vi "encoder_test_3mode_2motor_v2.vi"() -> ()   [LabVIEW 2014]
uses:
  <vilib>/eio/EIONode/EIONode.xnode
  <vilib>/rvi/FXPMathLib/FxpMul/XNode/nifxpmath_Multiplier.xnode
  <vilib>/rvi/FXPMathLib/sim/FxpSim.dll
  <vilib>/rvi/eio/common/nirviEmuTemplateMethod_errors.vi
  <vilib>/rvi/FXPMathLib/FxpSinAndCos/XNode/nifxpmath_SinAndCos.xnode
  <vilib>/rvi/FXPMathLib/FxpSinAndCos/simVIs/DllFxpSinAndCosTemp_sub.vi
  <vilib>/rvi/FXPMathLib/FxpSinAndCos/subVIs/nifxpmath_SinAndCos_SimConfig.ctl
  <vilib>/rvi/Analysis/measure/butterworth/XNode/niFpgaButterworthFilter.xnode
  <vilib>/rvi/FXPMathLib/FxpSub/XNode/nifxpmath_Sub.xnode
  <vilib>/rvi/FXPMathLib/FxpAdd/XNode/nifxpmath_Add.xnode
  <vilib>/rvi/DataTransferAndStorage/Container/XNode/niFpgaContainer.xnode
  <vilib>/rvi/interface/RandomDataEmulation/nirviRandomDataFpgaMultiElementTemplate.vi
panel:
  out "Dy_i":fxp<+/-,32,16>
  out "Dyr":fxp<+/-,64,32>
  in  "Direction_y":bool
  in  "Command type_y":i16(ring) items=["Step", "Ramp", "Sine"]
  out "Dy_error":fxp<+/-,57,33>
  out "Fmr_y":fxp<+/-,64,50>
  in  "Ki_y":fxp<+/-,16,1>
  in  "Dy_tolorence":fxp<+/-,18,1>
  in  "Kd_y":fxp<+/-,16,1>
  in  "Kp_y":fxp<+/-,16,1>
  in  "scaled coefficients_Dy_dd":i32[](array[numeric])=[780119100, 146811362]
  out "Dy_dd":fxp<+/-,36,47>
  out "va_y":fxp<+/-,36,7>
  out "vb_y":fxp<+/-,37,8>
  out "vd_y":fxp<+/-,20,5>
  out "vq_y":fxp<+/-,20,5> format="%.57g"
  in  "Stop motor_y":bool
  out "Dy_d (mm/s)":fxp<+,64,32>
  out "omega_y (rad/s)":fxp<+/-,64,35>
  in  "Velocity Estimation_y":i16(ring) items=["Step", "Ramp", "Sine"]
  out "Dy_d (T)":fxp<+/-,46,10>
  out "mt 2":u32
  out "omega_y (T)":fxp<+/-,20,9>
  out "omega_y (M)":fxp<+/-,64,30>
  out "Dy_d (M)":fxp<+/-,64,27>
  in  "Dy_d_M_Tc (mSec)":u32 format="%#_6f"
  out "omega_y(M_avg)":fxp<+/-,64,35>
  out "Dy_d (M_avg)":fxp<+,64,32>
  in  "Dy_d_M_avg_Tc (uSec)":u32 caption="Count(uSec)"
  out "rad_y(NrTheta)":fxp<+/-,48,33>
  out "Dy (mm)":fxp<+/-,56,32>
  out "Encoder Position_y":i32
  in  "Encoder Reset_y":bool
  out "omega_p (M_avg)":fxp<+/-,64,35>
  out "Dp_d (M_avg)":fxp<+/-,64,32>
  in  "Dp_d_M_avg_Tc (uSec)":u32 caption="D_d_M_avg_Tc (uSec)"
  out "omega_p (M)":fxp<+/-,64,30>
  out "Dp_d (M)":fxp<+/-,64,27>
  in  "Dp_d_M_Tc (mSec)":u32 format="%#_6f"
  out "Dp_d (T)":fxp<+/-,46,10>
  out "omega_p(T)":fxp<+/-,20,9>
  in  "Velocity Estimation_p":i16(ring) items=["M_avg method", "M method", "T method"]
  out "Dpr_ramp":fxp<+/-,64,30>
  out "Dpr_slope":fxp<+/-,33,17>
  in  "Dpr_time":fxp<+/-,16,11>
  out "Dpr_sin":fxp<+/-,28,11>
  out "Dpr_sin_d":fxp<+/-,64,16>
  out "Dpr_sin_dd":fxp<+/-,64,25>
  out "Sin omega_p":fxp<+/-,41,8>
  in  "Sin offset_p":fxp<+/-,27,10>
  in  "Sin magnitude_p":fxp<+/-,11,8>
  in  "Sin wave frequency_p (Hz)":fxp<+/-,21,5>
  out "Time now (s)":fxp<+,52,14>
  out "Dpr":fxp<+/-,64,31>
  in  "Dpr_end":fxp<+/-,16,11>
  in  "Command type_p":i16(ring) items=["Step", "Ramp", "Sine"]
  out "Dp_i":fxp<+/-,34,18>
  in  "Dp_tolorence":fxp<+/-,18,1>
  in  "Ki_p":fxp<+/-,20,6>
  out "Dp_error":fxp<+/-,24,11>
  in  "Direction_p":bool
  out "Fmr_p":fxp<+/-,64,31>
  in  "Kd_p":fxp<+/-,20,8>
  in  "Kp_p":fxp<+/-,20,12>
  in  "scaled coefficients_Dp_dd":i32[](array[numeric])=[780119100, 146811362]
  out "Dp_dd":fxp<+/-,36,29>
  in  "Ini coe.":bool
  out "va_p":fxp<+/-,38,8>
  out "vb_p":fxp<+/-,38,8>
  in  "Stop motor_p":bool
  out "vq_p":fxp<+/-,20,5> format="%.57g"
  out "vd_p":fxp<+/-,20,5>
  out "Dp_d (mm/s)":fxp<+/-,32,12>
  out "mt":u32
  out "omega_p (rad/s)":fxp<+/-,32,18>
  in  "mt0":u32
  out "Dp (mm)":fxp<+/-,22,7>
  out "rad_p(NrTheta)":fxp<+/-,33,18>
  out "Encoder Position_p":i32
  in  "Encoder Reset_p":bool
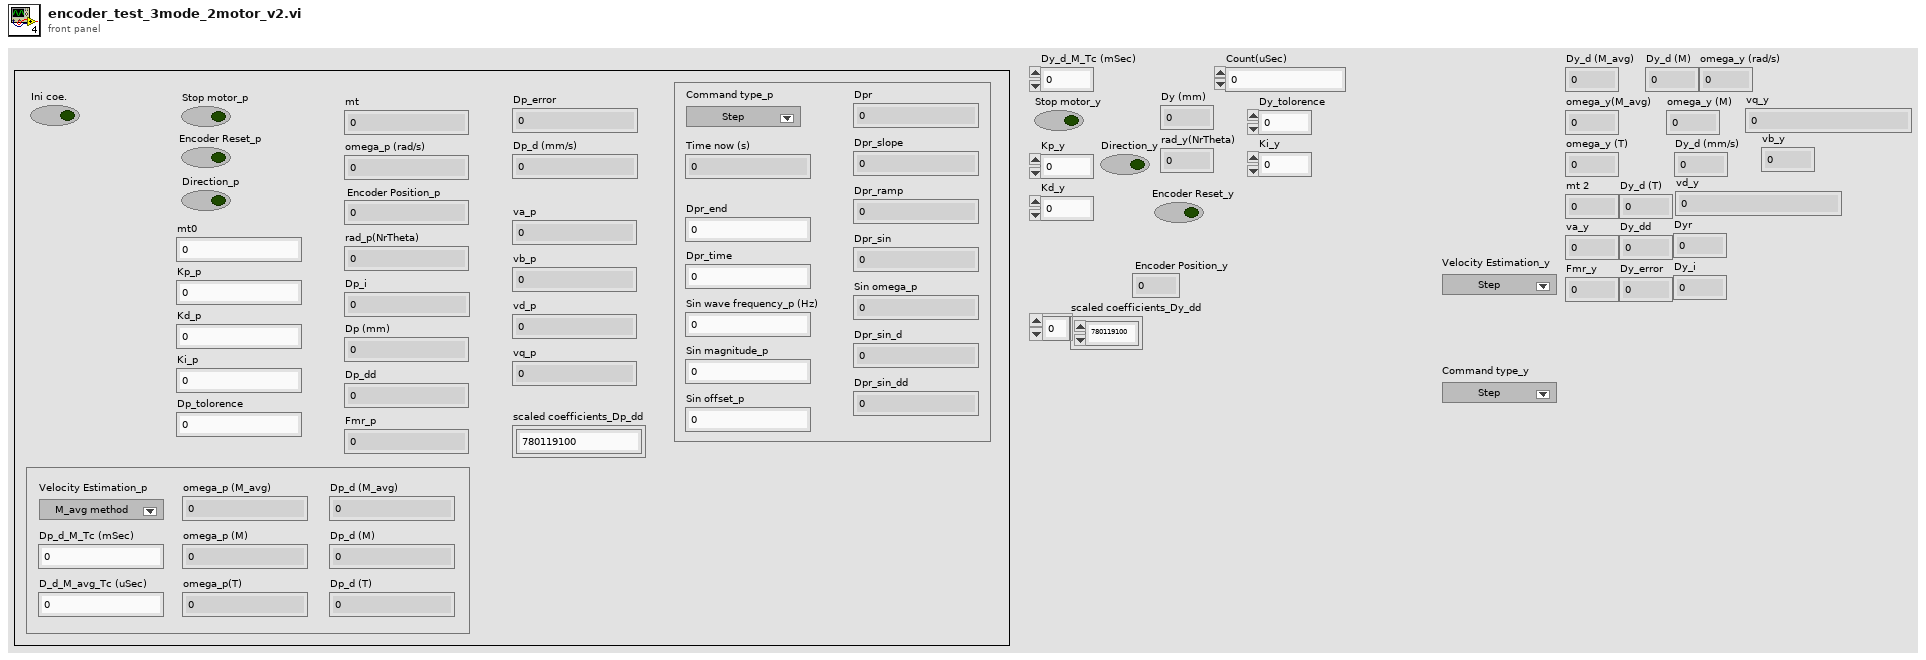
[diagram p1: front panel]
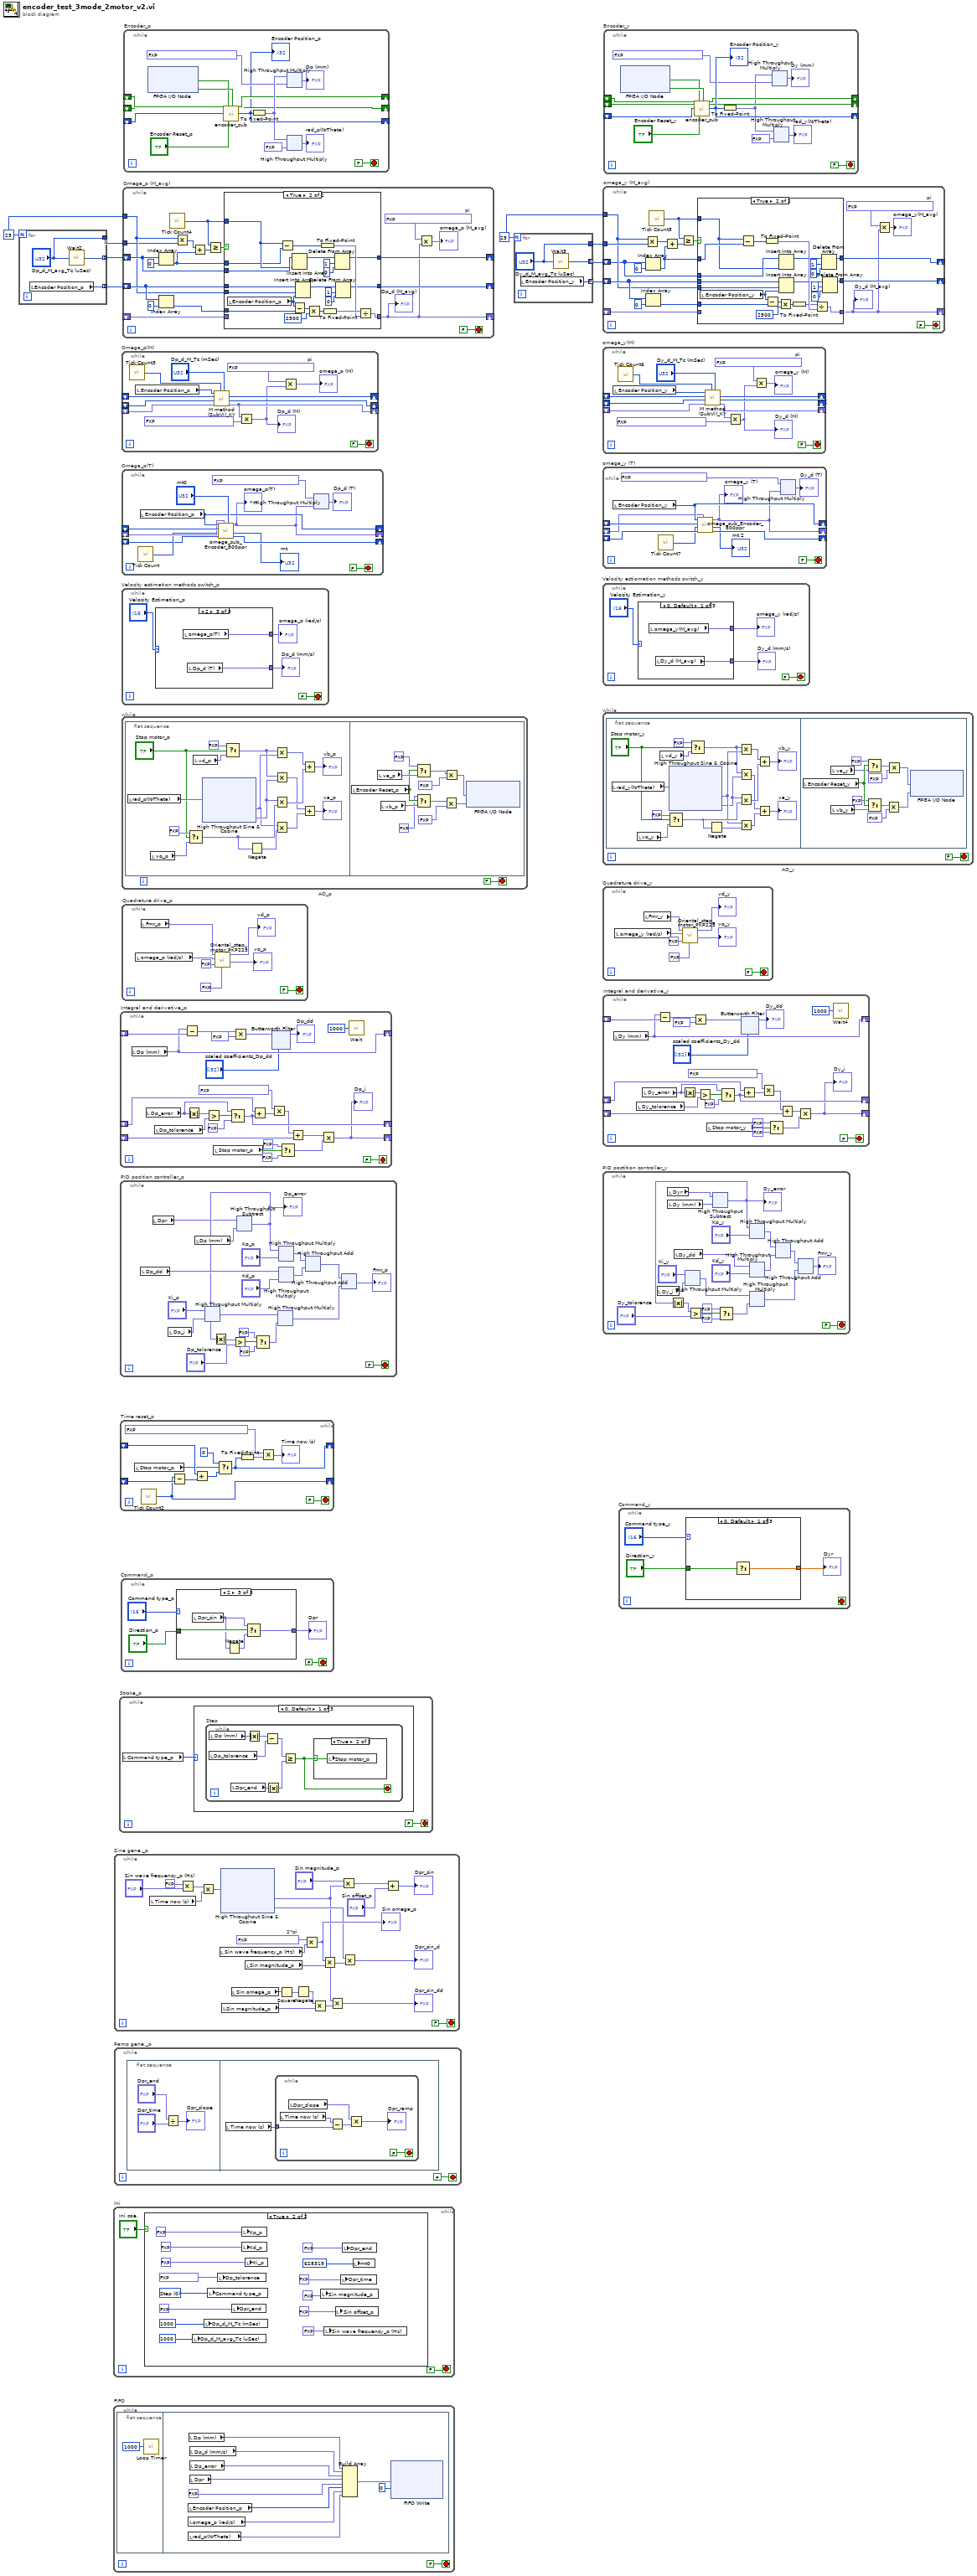
[diagram p0: block diagram]
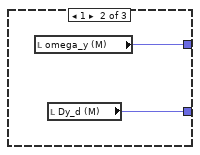
[diagram p4: hidden frame]
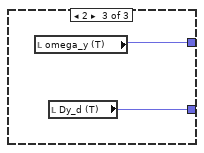
[diagram p5: hidden frame]
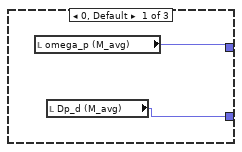
[diagram p8: hidden frame]
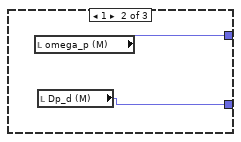
[diagram p9: hidden frame]
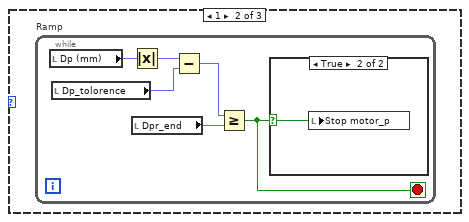
[diagram p11: hidden frame]
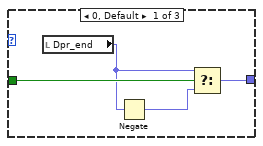
[diagram p14: hidden frame]
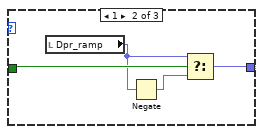
[diagram p15: hidden frame]
diagram:
  w4 = 25
  w8 = 25
  n1 = for {
    N: w8 -> [_]
    tunnel: ["Dp_d_M_avg_Tc (uSec)"] -> w5
    tunnel: [w10] -> w7 mode=indexing
    tunnel: [w9] -> w6 mode=indexing
    n2 = local read "Encoder Position_p"() -> (w9:i32)
    n3 = call "Wait2"("Count(uSec)"="Dp_d_M_avg_Tc (uSec)") -> ("Tick Count(uSec)"=w10:u32)
  }
  n4 = while "Ini" {
    stop <- FALSE stop-if-true
    n5 = case shown="True" "Ini coe." {
      frame False {
      }
      frame True {
        w21 = i16 0 items=["Step", "Ramp", "Sine"] ("Command type")
        n6 = local write "Dp_d_M_avg_Tc (uSec)"(u32 1000 ("D_d_M_avg_Tc (uSec)")) -> ()
        n7 = local write "Dp_d_M_Tc (mSec)"(u32 1000 ("D_d_M_Tc (uSec)")) -> ()
        n8 = local write "Command type_p"(w21) -> ()
        n9 = local write "Dp_tolorence"(fxp<+/-,14,3> 0.009765625 ("D_tolorence")) -> ()
        n10 = local write "Dpr_end"(fxp<+/-,16,11> 20.0 ("Dr_end")) -> ()
        n11 = local write "Kp_p"(fxp<+/-,20,12> 10.0 ("Kp")) -> ()
        n12 = local write "Kd_p"(fxp<+/-,20,8> 2.0 ("Kd")) -> ()
        n13 = local write "Ki_p"(fxp<+/-,20,6> 8.0 ("D_i")) -> ()
        n14 = local write "Sin magnitude_p"(fxp<+/-,11,8> 20.0 ("Sin magnitude")) -> ()
        n15 = local write "Sin wave frequency_p (Hz)"(fxp<+/-,21,5> 0.5 ("Sin wave frequency (Hz)")) -> ()
        n16 = local write "Sin offset_p"(fxp<+/-,27,10> 0.0 ("Sin offset")) -> ()
        n17 = local write "Dpr_time"(fxp<+/-,16,11> 5.0 ("Dr_time")) -> ()
        n18 = local write "Dpr_end"(fxp<+/-,11,7> 20.0 ("Fmr")) -> ()
        n19 = local write "mt0"(u32 628319 ("mt0")) -> ()
      }
    }
  }
  n20 = while "FIFO" {
    stop <- FALSE stop-if-true
    n21 = flat-sequence {
      frame #0 {
        n22 = call "Loop Timer"("Count(uSec)"=u32 1000) -> ()  [unwired: 1 out]
      }
      frame #1 {
        n23 = local read "Encoder Position_p"() -> (w33:i32)
        n24 = local read "omega_p (rad/s)"() -> (w32:fxp<+/-,32,18>)
        n25 = local read "rad_p(NrTheta)"() -> (w31:fxp<+/-,33,18>)
        n26 = local read "Dp (mm)"() -> (w37:fxp<+/-,22,7>)
        n27 = local read "Dp_d (mm/s)"() -> (w36:fxp<+/-,32,12>)
        n28 = local read "Dp_error"() -> (w35:fxp<+/-,24,11>)
        n29 = local read "Dpr"() -> (w34:fxp<+/-,64,31>)
        n30 = Build Array(w37, w36, w35, w34, fxp<+/-,64,32> 0.0 ("element"), w33, w32, w31) -> (w38:fxp<+/-,64,32>[])
        n31 = xnode ("FIFO Write")("Element"=w38, "Timeout"=0) -> ()  [unwired: 1 in, 2 out]
      }
    }
  }
  n32 = while "Sine gene._p" {
    stop <- FALSE stop-if-true
    w57 = fxp<+,20,3> 6.2831878662109375  # 2*pi
    n33 = local read "Time now (s)"() -> (w60:fxp<+,52,14>)
    n34 = Multiply(x=fxp<+,1,2> 2.0, y="Sin wave frequency_p (Hz)") -> (x*y=w61:fxp<+/-,21,6>)
    n35 = Multiply(x=w61, y=w60) -> (x*y=w41:fxp<+/-,64,20>)
    n36 = local read "Sin wave frequency_p (Hz)"() -> (w56:fxp<+/-,21,5>)
    n37 = xnode "High Throughput Sine & Cosine"("x (pi)"=w41) -> ("sin(x)"=w45:fxp<+/-,16,2>, "cos(x)"=w52:fxp<+/-,16,2>)
    n38 = local read "Sin magnitude_p"() -> (w47:fxp<+/-,11,8>)
    n39 = local read "Sin omega_p"() -> (w48:fxp<+/-,41,8>)
    n40 = local read "Sin magnitude_p"() -> (w51:fxp<+/-,11,8>)
    n41 = Square(x=w48) -> (x^2=w49:fxp<+,64,14>)
    n42 = Negate(x=w49) -> (-x=w46:fxp<+/-,64,15>)
    n43 = Multiply(x=w57, y=w56) -> (x*y=w53:fxp<+/-,41,8>)
    "Sin omega_p" <- w53
    n44 = Multiply(x=w46, y=w47) -> (x*y=w50:fxp<+/-,64,23>)
    n45 = Multiply(x=w53, y=w51) -> (x*y=w58:fxp<+/-,51,15>)
    n46 = Multiply(x=w45, y=w50) -> (x*y=→"Dpr_sin_dd":fxp<+/-,64,25>)
    n47 = Multiply(x="Sin magnitude_p", y=w45) -> (x*y=w59:fxp<+/-,27,10>)
    n48 = Multiply(x=w52, y=w58) -> (x*y=→"Dpr_sin_d":fxp<+/-,64,16>)
    n49 = Add(x=w59, y="Sin offset_p") -> (x+y=→"Dpr_sin":fxp<+/-,28,11>)
  }
  n50 = while "Ramp gene._p" {
    stop <- FALSE stop-if-true
    n51 = flat-sequence {
      frame #0 {
        n52 = Divide(x="Dpr_end", y="Dpr_time") -> (x/y=→"Dpr_slope":fxp<+/-,33,17>)
      }
      frame #1 {
        n53 = local read "Time now (s)"() -> (w98:fxp<+,52,14>)
        n54 = while {
          tunnel: w98 -> [w104]
          stop <- FALSE stop-if-true
          n55 = local read "Time now (s)"() -> (w101:fxp<+,52,14>)
          n56 = local read "Dpr_slope"() -> (w102:fxp<+/-,33,17>)
          n57 = Subtract(x=w101, y=w104) -> (x-y=w103:fxp<+/-,53,15>)
          n58 = Multiply(x=w102, y=w103) -> (x*y=→"Dpr_ramp":fxp<+/-,64,30>)
        }
      }
    }
  }
  n59 = while "Stroke_p" {
    stop <- FALSE stop-if-true
    n60 = local read "Command type_p"() -> (w106:i16)
    n61 = case shown="0, Default" w106 {
      frame 0, Default {
        n62 = while "Step" {
          stop <- w107 stop-if-true
          n63 = local read "Dp_tolorence"() -> (w109:fxp<+/-,18,1>)
          n64 = local read "Dp (mm)"() -> (w111:fxp<+/-,22,7>)
          n65 = local read "Dpr_end"() -> (w113:fxp<+/-,16,11>)
          n66 = Absolute Value(x=w111) -> (abs(x)=w110:fxp<+,22,7>)
          n67 = Subtract(x=w110, y=w109) -> (x-y=w108:fxp<+/-,25,8>)
          n68 = Absolute Value(x=w113) -> (abs(x)=w112:fxp<+,16,11>)
          n69 = Greater Or Equal?(x=w108, y=w112) -> (x >= y?=w107:bool)
          n70 = case shown="True" w107 {
            selector: w107 -> [_ w114]
            frame False {
            }
            frame True {
              n71 = local write "Stop motor_p"(w114) -> ()
            }
          }
        }
      }
      frame 1 {
        n72 = while "Ramp" {
          stop <- w115 stop-if-true
          n73 = local read "Dp (mm)"() -> (w117:fxp<+/-,22,7>)
          n74 = local read "Dp_tolorence"() -> (w119:fxp<+/-,18,1>)
          n75 = Absolute Value(x=w117) -> (abs(x)=w118:fxp<+,22,7>)
          n76 = local read "Dpr_end"() -> (w116:fxp<+/-,16,11>)
          n77 = Subtract(x=w118, y=w119) -> (x-y=w120:fxp<+/-,25,8>)
          n78 = Greater Or Equal?(x=w120, y=w116) -> (x >= y?=w115:bool)
          n79 = case shown="True" w115 {
            selector: w115 -> [_ w121]
            frame False {
            }
            frame True {
              n80 = local write "Stop motor_p"(w121) -> ()
            }
          }
        }
      }
      frame 2 {
      }
    }
  }
  n81 = while "Integral and derivative_p" {
    shift-right: [w142] -> _
    shift-left: _ -> [w146]
    shift-right: [w132] -> _
    shift-left: _ -> [w133]
    shift-right: [w122] -> _
    shift-left: _ -> [w126]
    stop <- FALSE stop-if-true
    n82 = local read "Dp (mm)"() -> (w142:fxp<+/-,22,7>)
    n83 = local read "Dp_error"() -> (w134:fxp<+/-,24,11>)
    n84 = local read "Dp_tolorence"() -> (w137:fxp<+/-,18,1>)
    n85 = Subtract(x=w142, y=w146) -> (x-y=w145:fxp<+/-,23,8>)
    n86 = Absolute Value(x=w134) -> (abs(x)=w138:fxp<+,24,11>)
    n87 = Greater?(x=w138, y=w137) -> (0:w136:bool)
    n88 = local read "Stop motor_p"() -> (w129:bool)
    n89 = Select(t=w134, s=w136, f=fxp<+,24,11> 0.0) -> (s? t:f=w132:fxp<+/-,25,12>)
    n90 = Multiply(x=w145, y=fxp<+/-,33,13> 1000.0) -> (x*y=w143:fxp<+/-,55,20>)
    n91 = Add(x=w133, y=w132) -> (x+y=w131:fxp<+/-,26,13>)
    n92 = Multiply(x=fxp<+/-,30,12> 0.000499725341796875, y=w131) -> (x*y=w125:fxp<+/-,55,24>)
    n93 = xnode "Butterworth Filter"("input data"=w143, "scaled coefficients"="scaled coefficients_Dp_dd") -> ("output data"=→"Dp_dd":fxp<+/-,36,24>)  [unwired: 1 in]
    n94 = Select(t=fxp<+,1,1> 0.0, s=w129, f=fxp<+,1,1> 1.0) -> (s? t:f=w123:fxp<+,1,1>)
    n95 = Add(x=w125, y=w126) -> (x+y=w124:fxp<+/-,32,16>)
    n96 = Multiply(x=w124, y=w123) -> (x*y=w122:fxp<+/-,32,16>)
    "Dp_i" <- w122
    n97 = call "Wait"("Count(uSec)"=u32 1000) -> ()  [unwired: 1 out]
  }
  n98 = while "PID position controller_p" {
    stop <- FALSE stop-if-true
    n99 = local read "Dp_dd"() -> (w172:fxp<+/-,36,29>)
    n100 = local read "Dpr"() -> (w156:fxp<+/-,64,31>)
    n101 = local read "Dp_i"() -> (w167:fxp<+/-,34,18>)
    n102 = local read "Dp (mm)"() -> (w176:fxp<+/-,22,7>)
    n103 = xnode ("High Throughput Multiply")("x"="Ki_p", "y"=w167) -> ("x*y"=w161:fxp<+/-,54,24>)
    n104 = xnode "High Throughput Subtract"("x"=w156, "y"=w176) -> ("x-y"=w165:fxp<+/-,64,32>)
    "Dp_error" <- w165
    n105 = Absolute Value(x=w165) -> (abs(x)=w166:fxp<+,64,32>)
    n106 = Greater?(x=w166, y="Dp_tolorence") -> (0:w164:bool)
    n107 = Select(t=fxp<+,10,2> 1.0, s=w164, f=fxp<+,10,2> 0.0) -> (s? t:f=w160:fxp<+,10,2>)
    n108 = xnode ("High Throughput Multiply")("x"=w161, "y"=w160) -> ("x*y"=w157:fxp<+/-,64,26>)
    n109 = xnode ("High Throughput Multiply")("x"=w165, "y"="Kp_p") -> ("x*y"=w174:fxp<+/-,64,44>)
    n110 = xnode ("High Throughput Multiply")("x"=w172, "y"="Kd_p") -> ("x*y"=w173:fxp<+/-,56,37>)
    n111 = xnode ("High Throughput Add")("x"=w174, "y"=w173) -> ("x+y"=w158:fxp<+/-,64,45>)
    n112 = xnode ("High Throughput Add")("x"=w158, "y"=w157) -> ("x+y"=→"Fmr_p":fxp<+/-,64,46>)
  }
  n113 = while "Time reset_p" {
    shift-right: [w180] -> _
    shift-left: _ -> [w187]
    shift-right: [w182] -> _
    shift-left: _ -> [w183]
    stop <- FALSE stop-if-true
    n114 = local read "Stop motor_p"() -> (w185:bool)
    n115 = call "Tick Count2"() -> ("Tick Count(uSec)"=w182:u32)
    n116 = Subtract(x=w182, y=w183) -> (x-y=w188:u32)
    n117 = Add(x=w187, y=w188) -> (x+y=w186:u32)
    n118 = Select(t=u32 0, s=w185, f=w186) -> (s? t:f=w180:u32)
    n119 = To Fixed-Point(number=w180) -> (fixed-point=w179:fxp<+,32,32>)  [unwired: 1 in]
    n120 = Multiply(x=fxp<+,20,-18> 1.0000003385357559e-06, y=w179) -> (x*y=→"Time now (s)":fxp<+,52,14>)
  }
  n121 = while "Command_p" {
    stop <- FALSE stop-if-true
    n122 = case shown="2" "Command type_p" {
      tunnel: [w193 w197 w201] -> w191
      tunnel: "Direction_p" -> [w196 w200 w204]
      frame 0, Default {
        n123 = local read "Dpr_end"() -> (w195:fxp<+/-,16,11>)
        n124 = Negate(x=w195) -> (-x=w194:fxp<+/-,17,12>)
        n125 = Select(t=w195, s=w196, f=w194) -> (s? t:f=w193:fxp<+/-,17,12>)
      }
      frame 1 {
        n126 = local read "Dpr_ramp"() -> (w198:fxp<+/-,64,30>)
        n127 = Negate(x=w198) -> (-x=w199:fxp<+/-,64,31>)
        n128 = Select(t=w198, s=w200, f=w199) -> (s? t:f=w197:fxp<+/-,64,31>)
      }
      frame 2 {
        n129 = local read "Dpr_sin"() -> (w202:fxp<+/-,28,11>)
        n130 = Negate(x=w202) -> (-x=w203:fxp<+/-,27,10>)
        n131 = Select(t=w202, s=w204, f=w203) -> (s? t:f=w201:fxp<+/-,28,11>)
      }
    }
    "Dpr" <- w191
  }
  n132 = while "Omega_p(M)" {
    shift-right: [w216] -> _
    shift-left: _ -> [w217]
    shift-right: [w212] -> _
    shift-left: _ -> [w213]
    shift-right: [w210] -> _
    shift-left: _ -> [w211]
    stop <- FALSE stop-if-true
    w207 = fxp<+/-,27,3> 3.1415926218032837  # pi
    n133 = call "Tick Count3"() -> ("Tick Count(mSec)"=w215:u32)
    n134 = local read "Encoder Position_p"() -> (w218:i32)
    n135 = call "M method (SubVI)_KY.vi"("Tc (mSec)"="Dp_d_M_Tc (mSec)", "Tick Count (mSec)"=w215, "Encoder velocity_pre (pulse/s)"=w211, "Shift Register in 2"=w213, "Shift Register in 1"=w217, "Encoder pulses"=w218) -> ("Encoder velocity (pulse/s)"=w210:fxp<+/-,64,32>, "Shift Register out 2"=w212:i32, "Shift Register out 1"=w216:u32)  [unwired: 3 in]
    n136 = Multiply(x=w210, y=fxp<+/-,20,-5> 0.002499997615814209) -> (x*y=w208:fxp<+/-,64,27>)
    "Dp_d (M)" <- w208
    n137 = Multiply(x=w207, y=w208) -> (x*y=→"omega_p (M)":fxp<+/-,64,30>)
  }
  n138 = while "Omega_p(T)" {
    shift-right: [w228] -> _
    shift-left: _ -> [w229]
    shift-right: [w221] -> _
    shift-left: _ -> [w227]
    shift-right: [w224] -> _
    shift-left: _ -> [w225]
    stop <- FALSE stop-if-true
    n139 = call "Tick Count"() -> ("Tick Count(Ticks)"=w226:u32)
    n140 = local read "Encoder Position_p"() -> (w228:i32)
    n141 = call "omega_sub_Encoder_800ppr.vi"("mt0"="mt0", "omega_pre"=w227, "ticks_m_pre"=w225, "ticks"=w226, "count_pre"=w229, "count"=w228) -> ("ticks_m"=w224:u32, "mt"=→"mt":u32, "omega"=w221:fxp<+/-,20,9>)  [unwired: 3 in]
    "omega_p(T)" <- w221
    n142 = xnode ("High Throughput Multiply")("x"=fxp<+/-,26,1> 0.3183099031448364, "y"=w221) -> ("x*y"=→"Dp_d (T)":fxp<+/-,46,10>)
  }
  n143 = while "Velocity estimation methods switch_p" {
    stop <- FALSE stop-if-true
    n144 = case shown="2" "Velocity Estimation_p" {
      tunnel: [w236 w238 w240] -> w233
      tunnel: [w235 w237 w239] -> w232
      frame 0, Default {
        n145 = local read "omega_p (M_avg)"() -> (w236:fxp<+/-,64,35>)
        n146 = local read "Dp_d (M_avg)"() -> (w235:fxp<+/-,64,32>)
      }
      frame 1 {
        n147 = local read "omega_p (M)"() -> (w238:fxp<+/-,64,30>)
        n148 = local read "Dp_d (M)"() -> (w237:fxp<+/-,64,27>)
      }
      frame 2 {
        n149 = local read "omega_p(T)"() -> (w240:fxp<+/-,20,9>)
        n150 = local read "Dp_d (T)"() -> (w239:fxp<+/-,46,10>)
      }
    }
    "Dp_d (mm/s)" <- w232
    "omega_p (rad/s)" <- w233
  }
  n151 = while "AO_p" {
    stop <- FALSE stop-if-true
    n152 = flat-sequence {
      frame #0 {
        n153 = local read "rad_p(NrTheta)"() -> (w257:fxp<+/-,33,18>)
        n154 = local read "vq_p"() -> (w255:fxp<+/-,20,5>)
        n155 = Select(t=fxp<+,20,5> 0.0, s="Stop motor_p", f=w255) -> (s? t:f=w252:fxp<+/-,21,6>)
        n156 = local read "vd_p"() -> (w256:fxp<+/-,20,5>)
        n157 = xnode "High Throughput Sine & Cosine"("x (pi)"=w257) -> ("sin(x)"=w248:fxp<+/-,17,2>, "cos(x)"=w250:fxp<+/-,17,2>)
        n158 = Select(t=fxp<+,20,5> 0.0, s="Stop motor_p", f=w256) -> (s? t:f=w249:fxp<+/-,21,6>)
        n159 = Negate(x=w252) -> (-x=w251:fxp<+/-,21,6>)
        n160 = Multiply(x=w249, y=w248) -> (x*y=w247:fxp<+/-,37,7>)
        n161 = Multiply(x=w249, y=w250) -> (x*y=w245:fxp<+/-,37,7>)
        n162 = Multiply(x=w250, y=w252) -> (x*y=w246:fxp<+/-,37,7>)
        n163 = Multiply(x=w248, y=w251) -> (x*y=w244:fxp<+/-,37,7>)
        n164 = Add(x=w247, y=w246) -> (x+y=→"vb_p":fxp<+/-,38,8>)
        n165 = Add(x=w245, y=w244) -> (x+y=→"va_p":fxp<+/-,38,8>)
      }
      frame #1 {
        n166 = local read "Encoder Reset_p"() -> (w291:bool)
        n167 = local read "va_p"() -> (w293:fxp<+/-,38,8>)
        n168 = local read "vb_p"() -> (w292:fxp<+/-,38,8>)
        n169 = Select(t=fxp<+/-,20,5> 5.0 ("y"), s=w291, f=w293) -> (s? t:f=w294:fxp<+/-,38,8>)
        n170 = Select(t=fxp<+/-,20,5> 0.0 ("y"), s=w291, f=w292) -> (s? t:f=w295:fxp<+/-,38,8>)
        n171 = Multiply(x=w295, y=fxp<+/-,20,5> -0.5) -> (x*y=w299:fxp<+/-,57,12>)
        n172 = Multiply(x=w294, y=fxp<+/-,20,5> -0.5) -> (x*y=w298:fxp<+/-,57,12>)
        n173 = xnode "FPGA I/O Node"("Mod8/AO0"=w298, "Mod8/AO1"=w299) -> ()  [unwired: 2 in, 2 out]
      }
    }
  }
  n174 = while "Quadrature drive_p" {
    stop <- FALSE stop-if-true
    n175 = local read "omega_p (rad/s)"() -> (w302:fxp<+/-,32,18>)
    n176 = local read "Fmr_p"() -> (w300:fxp<+/-,64,31>)
    n177 = call "Oriental_step_motor_PKP225.vi"("F_Threshold"=fxp<+,12,12> 10.0, "dFmr"=fxp<+/-,25,15> 0.0, "omega"=w302, "Fmr"=w300) -> ("vq_F"=→"vq_p":fxp<+/-,20,5>, "vd_F"=→"vd_p":fxp<+/-,20,5>)  [unwired: 6 in]
  }
  n178 = while "Omega_p (M_avg)" {
    tunnel: w8 -> [w318]
    shift-right: [w311] -> _
    shift-left: w7 -> [w322]
    shift-right: [w310] -> _
    shift-left: _ -> [w313]
    shift-right: [w312] -> _
    shift-left: w6 -> [w321]
    tunnel: w5 -> [w315]
    stop <- FALSE stop-if-true
    w309 = fxp<+/-,27,3> 3.1415926218032837  # pi
    n179 = Index Array(array=w322, index=0) -> (element=w316:u32)
    n180 = Index Array(array=w321, index=0) -> (element=w317:i32)
    n181 = call "Tick Count4"() -> ("Tick Count(uSec)"=w319:u32)
    n182 = Multiply(x=w318, y=w315) -> (x*y=w323:u32)
    n183 = Add(x=w323, y=w316) -> (x+y=w320:u32)
    n184 = Greater Or Equal?(x=w319, y=w320) -> (x >= y?=w314:bool)
    n185 = case shown="True" w314 {
      tunnel: w322 -> [w328 w345]
      tunnel: w321 -> [w327 w344]
      tunnel: w319 -> [_ w337]
      tunnel: w318 -> [_ w343]
      tunnel: w317 -> [_ w341]
      tunnel: w316 -> [_ w336]
      tunnel: w313 -> [w326 _]
      tunnel: [w327 w331] -> w312
      tunnel: [w328 w330] -> w311
      tunnel: [w326 w329] -> w310
      frame False {
      }
      frame True {
        n186 = local read "Encoder Position_p"() -> (w342:i32)
        n187 = Subtract(x=w337, y=w336) -> (x-y=w334:u32)
        n188 = Insert Into Array(array=w345, new element=w337) -> (w346:u32[])  [unwired: 1 in]
        n189 = Subtract(x=w342, y=w341) -> (x-y=w340:i32)
        n190 = Insert Into Array(array=w344, index=w343, new element=w342) -> (w347:i32[])
        n191 = Multiply(x=w340, y=2500) -> (x*y=w338:i32)
        n192 = To Fixed-Point(number=w334) -> (fixed-point=w332:fxp<+,32,32>)  [unwired: 1 in]
        n193 = To Fixed-Point(number=w338) -> (fixed-point=w333:fxp<+/-,32,32>)  [unwired: 1 in]
        n194 = Delete From Array(array=w346, length=1, index=0) -> (array with subset deleted=w330:u32[])  [unwired: 1 out]
        n195 = Delete From Array(array=w347, length=1, index=0) -> (array with subset deleted=w331:i32[])  [unwired: 1 out]
        n196 = Divide(x=w333, y=w332) -> (x/y=w329:fxp<+/-,64,32>)
      }
    }
    "Dp_d (M_avg)" <- w310
    n197 = Multiply(x=w309, y=w310) -> (x*y=→"omega_p (M_avg)":fxp<+/-,64,35>)
  }
  n198 = while "Encoder_p" {
    shift-right: [w357] -> _
    shift-left: _ -> [w359]
    shift-right: [w356] -> _
    shift-left: _ -> [w358]
    shift-right: [w354] -> _
    shift-left: _ -> [w355]
    stop <- FALSE stop-if-true
    n199 = xnode "FPGA I/O Node"() -> ("Mod4/DI3"=w364:bool, "Mod4/DI4"=w365:bool)  [unwired: 2 in, 2 out]
    n200 = call "encoder_sub.vi"("A_pre"=w359, "B_pre"=w358, "Encoder Position_pre"=w355, "A input"=w364, "Encoder Position Reset"="Encoder Reset_p", "B input"=w365) -> ("A"=w357:bool, "B"=w356:bool, "Encoder Position (Counts)"=w354:i32)  [unwired: 19 in]
    "Encoder Position_p" <- w354
    n201 = To Fixed-Point(number=w354) -> (fixed-point=w362:fxp<+/-,32,32>)  [unwired: 1 in]
    n202 = xnode ("High Throughput Multiply")("x"=w362, "y"=fxp<+/-,24,0> 0.002499997615814209) -> ("x*y"=→"Dp (mm)":fxp<+/-,56,32>)
    n203 = xnode ("High Throughput Multiply")("x"=w362, "y"=fxp<+/-,24,0> 0.125) -> ("x*y"=→"rad_p(NrTheta)":fxp<+/-,56,32>)
  }
  n204 = for {
    N: w4 -> [_]
    tunnel: ["Dy_d_M_avg_Tc (uSec)"] -> w3
    tunnel: [w367] -> w1 mode=indexing
    tunnel: [w366] -> w2 mode=indexing
    n205 = local read "Encoder Position_y"() -> (w366:i32)
    n206 = call "Wait3"("Count(uSec)"="Dy_d_M_avg_Tc (uSec)") -> ("Tick Count(uSec)"=w367:u32)
  }
  n207 = while "omega_y(M)" {
    shift-right: [w375] -> _
    shift-left: _ -> [w379]
    shift-right: [w376] -> _
    shift-left: _ -> [w378]
    shift-right: [w374] -> _
    shift-left: _ -> [w377]
    stop <- FALSE stop-if-true
    w371 = fxp<+/-,27,3> 3.1415926218032837  # pi
    n208 = local read "Encoder Position_y"() -> (w382:i32)
    n209 = call "Tick Count6"() -> ("Tick Count(mSec)"=w381:u32)
    n210 = call "M method (SubVI)_KY.vi"("Tc (mSec)"="Dy_d_M_Tc (mSec)", "Tick Count (mSec)"=w381, "Encoder velocity_pre (pulse/s)"=w377, "Shift Register in 2"=w378, "Shift Register in 1"=w379, "Encoder pulses"=w382) -> ("Encoder velocity (pulse/s)"=w374:fxp<+/-,64,32>, "Shift Register out 2"=w376:i32, "Shift Register out 1"=w375:u32)  [unwired: 3 in]
    n211 = Multiply(x=w374, y=fxp<+/-,20,-5> 0.002499997615814209) -> (x*y=w372:fxp<+/-,64,27>)
    "Dy_d (M)" <- w372
    n212 = Multiply(x=w371, y=w372) -> (x*y=→"omega_y (M)":fxp<+/-,64,30>)
  }
  n213 = while "omega_y (T)" {
    shift-right: [w392] -> _
    shift-left: _ -> [w391]
    shift-right: [w386] -> _
    shift-left: _ -> [w390]
    shift-right: [w393] -> _
    shift-left: _ -> [w389]
    stop <- FALSE stop-if-true
    n214 = local read "Encoder Position_y"() -> (w392:i32)
    n215 = call "Tick Count7"() -> ("Tick Count(Ticks)"=w388:u32)
    n216 = call "omega_sub_Encoder_800ppr.vi"("omega_pre"=w390, "ticks_m_pre"=w389, "ticks"=w388, "count_pre"=w391, "count"=w392) -> ("ticks_m"=w393:u32, "mt"=→"mt 2":u32, "omega"=w386:fxp<+/-,20,9>)  [unwired: 4 in]
    "omega_y (T)" <- w386
    n217 = xnode "High Throughput Multiply"("x"=fxp<+/-,26,1> 0.3183099031448364, "y"=w386) -> ("x*y"=→"Dy_d (T)":fxp<+/-,46,10>)
  }
  n218 = while "Velocity estiomation methods switch_y" {
    stop <- FALSE stop-if-true
    n219 = case shown="0, Default" "Velocity Estimation_y" {
      tunnel: [w399 w400 w403] -> w396
      tunnel: [w398 w401 w402] -> w395
      frame 0, Default {
        n220 = local read "omega_y(M_avg)"() -> (w399:fxp<+/-,64,35>)
        n221 = local read "Dy_d (M_avg)"() -> (w398:fxp<+,64,32>)
      }
      frame 1 {
        n222 = local read "omega_y (M)"() -> (w400:fxp<+/-,64,30>)
        n223 = local read "Dy_d (M)"() -> (w401:fxp<+/-,64,27>)
      }
      frame 2 {
        n224 = local read "omega_y (T)"() -> (w403:fxp<+/-,20,9>)
        n225 = local read "Dy_d (T)"() -> (w402:fxp<+/-,46,10>)
      }
    }
    "omega_y (rad/s)" <- w396
    "Dy_d (mm/s)" <- w395
  }
  n226 = while "AO_y" {
    stop <- FALSE stop-if-true
    n227 = flat-sequence {
      frame #0 {
        n228 = local read "rad_y(NrTheta)"() -> (w416:fxp<+/-,48,33>)
        n229 = local read "vq_y"() -> (w419:fxp<+/-,20,5>)
        n230 = local read "vd_y"() -> (w418:fxp<+/-,20,5>)
        n231 = xnode "High Throughput Sine & Cosine"("x (pi)"=w416) -> ("sin(x)"=w412:fxp<+/-,16,2>, "cos(x)"=w411:fxp<+/-,16,2>)
        n232 = Select(t=fxp<+,1,1> 0.0, s="Stop motor_y", f=w419) -> (s? t:f=w414:fxp<+/-,20,5>)
        n233 = Select(t=fxp<+/-,20,5> 0.0, s="Stop motor_y", f=w418) -> (s? t:f=w413:fxp<+/-,20,5>)
        n234 = Negate(x=w414) -> (-x=w415:fxp<+/-,21,6>)
        n235 = Multiply(x=w413, y=w412) -> (x*y=w410:fxp<+/-,36,7>)
        n236 = Multiply(x=w413, y=w411) -> (x*y=w408:fxp<+/-,36,7>)
        n237 = Multiply(x=w411, y=w414) -> (x*y=w409:fxp<+/-,36,7>)
        n238 = Multiply(x=w412, y=w415) -> (x*y=w407:fxp<+/-,35,6>)
        n239 = Add(x=w410, y=w409) -> (x+y=→"vb_y":fxp<+/-,37,8>)
        n240 = Add(x=w408, y=w407) -> (x+y=→"va_y":fxp<+/-,36,7>)
      }
      frame #1 {
        n241 = local read "Encoder Reset_y"() -> (w462:bool)
        n242 = local read "va_y"() -> (w461:fxp<+/-,36,7>)
        n243 = local read "vb_y"() -> (w460:fxp<+/-,37,8>)
        n244 = Select(t=fxp<+/-,20,5> 5.0, s=w462, f=w461) -> (s? t:f=w457:fxp<+/-,36,7>)
        n245 = Select(t=fxp<+/-,20,5> 0.0, s=w462, f=w460) -> (s? t:f=w456:fxp<+/-,37,8>)
        n246 = Multiply(x=w456, y=fxp<+/-,20,5> -0.5) -> (x*y=w452:fxp<+/-,55,11>)
        n247 = Multiply(x=w457, y=fxp<+/-,20,5> -0.5) -> (x*y=w453:fxp<+/-,55,11>)
        n248 = xnode "FPGA I/O Node"("Mod8/AO2"=w453, "Mod8/AO3"=w452) -> ()  [unwired: 2 in, 2 out]
      }
    }
  }
  n249 = while "Quadrature drive_y" {
    stop <- FALSE stop-if-true
    n250 = local read "omega_y (rad/s)"() -> (w469:fxp<+/-,64,35>)
    n251 = local read "Fmr_y"() -> (w464:fxp<+/-,64,50>)
    n252 = call "Oriental_step_motor_PKP225.vi"("F_Threshold"=fxp<+,12,12> 10.0, "dFmr"=fxp<+/-,25,15> 0.0, "omega"=w469, "Fmr"=w464) -> ("vq_F"=→"vq_y":fxp<+/-,20,5>, "vd_F"=→"vd_y":fxp<+/-,20,5>)  [unwired: 6 in]
  }
  n253 = while "PID postition controller_y" {
    stop <- FALSE stop-if-true
    n254 = local read "Dy_i"() -> (w471:fxp<+/-,32,16>)
    n255 = local read "Dyr"() -> (w472:fxp<+/-,64,32>)
    n256 = local read "Dy (mm)"() -> (w481:fxp<+/-,56,32>)
    n257 = local read "Dy_dd"() -> (w482:fxp<+/-,36,47>)
    n258 = xnode "High Throughput Multiply"("x"="Ki_y", "y"=w471) -> ("x*y"=w480:fxp<+/-,48,17>)
    n259 = xnode "High Throughput Subtract"("x"=w472, "y"=w481) -> ("x-y"=w473:fxp<+/-,64,33>)
    "Dy_error" <- w473
    n260 = Absolute Value(x=w473) -> (abs(x)=w474:fxp<+,64,33>)
    n261 = Greater?(x=w474, y="Dy_tolorence") -> (0:w485:bool)
    n262 = Select(t=fxp<+,1,1> 1.0, s=w485, f=fxp<+,1,1> 0.0) -> (s? t:f=w488:fxp<+,1,1>)
    n263 = xnode "High Throughput Multiply"("x"=w473, "y"="Kp_y") -> ("x*y"=w479:fxp<+/-,64,34>)
    n264 = xnode "High Throughput Multiply"("x"=w482, "y"="Kd_y") -> ("x*y"=w478:fxp<+/-,52,48>)
    n265 = xnode "High Throughput Multiply"("x"=w480, "y"=w488) -> ("x*y"=w476:fxp<+/-,48,17>)
    n266 = xnode "High Throughput Add"("x"=w479, "y"=w478) -> ("x+y"=w477:fxp<+/-,64,49>)
    n267 = xnode "High Throughput Add"("x"=w477, "y"=w476) -> ("x+y"=→"Fmr_y":fxp<+/-,64,50>)
  }
  n268 = while "omega_y (M_avg)" {
    tunnel: w4 -> [w500]
    tunnel: w3 -> [w506]
    shift-right: [w496] -> _
    shift-left: w1 -> [w497]
    shift-right: [w495] -> _
    shift-left: w2 -> [w501]
    shift-right: [w493] -> _
    shift-left: _ -> [w498]
    stop <- FALSE stop-if-true
    w494 = fxp<+/-,27,3> 3.1415926218032837  # pi
    n269 = Multiply(x=w500, y=w506) -> (x*y=w505:u32)
    n270 = Index Array(array=w497, index=0) -> (element=w502:u32)
    n271 = Index Array(array=w501, index=0) -> (element=w499:i32)
    n272 = call "Tick Count5"() -> ("Tick Count(uSec)"=w503:u32)
    n273 = Add(x=w505, y=w502) -> (x+y=w509:u32)
    n274 = Greater Or Equal?(x=w503, y=w509) -> (x >= y?=w504:bool)
    n275 = case shown="True" w504 {
      tunnel: w503 -> [_ w532]
      tunnel: w502 -> [_ w533]
      tunnel: w501 -> [w511 w522]
      tunnel: w500 -> [_ w523]
      tunnel: w499 -> [_ w524]
      tunnel: w498 -> [w510 _]
      tunnel: w497 -> [w512 w534]
      tunnel: [w512 w515] -> w496
      tunnel: [w511 w514] -> w495
      tunnel: [w510 w513] -> w493
      frame False {
      }
      frame True {
        n276 = local read "Encoder Position_y"() -> (w525:i32)
        n277 = Subtract(x=w532, y=w533) -> (x-y=w531:u32)
        n278 = To Fixed-Point(number=w531) -> (fixed-point=w530:fxp<+,32,32>)  [unwired: 1 in]
        n279 = Subtract(x=w525, y=w524) -> (x-y=w526:i32)
        n280 = Multiply(x=w526, y=u32 2500) -> (x*y=w528:u32)
        n281 = Insert Into Array(array=w534, new element=w532) -> (w520:u32[])  [unwired: 1 in]
        n282 = Insert Into Array(array=w522, index=w523, new element=w525) -> (w521:i32[])
        n283 = To Fixed-Point(number=w528) -> (fixed-point=w529:fxp<+,32,32>)  [unwired: 1 in]
        n284 = Divide(x=w529, y=w530) -> (x/y=w513:fxp<+,64,32>)
        n285 = Delete From Array(array=w520, length=1, index=0) -> (array with subset deleted=w515:u32[])  [unwired: 1 out]
        n286 = Delete From Array(array=w521, length=1, index=0) -> (array with subset deleted=w514:i32[])  [unwired: 1 out]
      }
    }
    "Dy_d (M_avg)" <- w493
    n287 = Multiply(x=w494, y=w493) -> (x*y=→"omega_y(M_avg)":fxp<+/-,64,35>)
  }
  n288 = while "Integral and derivative_y" {
    shift-right: [w556] -> _
    shift-left: _ -> [w559]
    shift-right: [w545] -> _
    shift-left: _ -> [w536]
    shift-right: [w538] -> _
    shift-left: _ -> [w537]
    stop <- FALSE stop-if-true
    n289 = local read "Dy (mm)"() -> (w556:fxp<+/-,56,32>)
    n290 = local read "Dy_tolorence"() -> (w551:fxp<+/-,18,1>)
    n291 = local read "Dy_error"() -> (w548:fxp<+/-,57,33>)
    n292 = Subtract(x=w556, y=w559) -> (x-y=w558:fxp<+/-,57,33>)
    n293 = Absolute Value(x=w548) -> (abs(x)=w552:fxp<+,57,33>)
    n294 = Multiply(x=w558, y=fxp<+,7,10> 1000.0) -> (x*y=w555:fxp<+/-,64,43>)
    n295 = Greater?(x=w552, y=w551) -> (0:w550:bool)
    n296 = local read "Stop motor_y"() -> (w542:bool)
    n297 = Select(t=w548, s=w550, f=fxp<+,24,11> 0.0) -> (s? t:f=w545:fxp<+/-,57,33>)
    n298 = xnode "Butterworth Filter"("input data"=w555, "scaled coefficients"="scaled coefficients_Dy_dd") -> ("output data"=→"Dy_dd":fxp<+/-,36,47>)  [unwired: 1 in]
    n299 = Add(x=w536, y=w545) -> (x+y=w547:fxp<+/-,58,34>)
    n300 = Multiply(x=fxp<+/-,30,12> 0.000499725341796875, y=w547) -> (x*y=w544:fxp<+/-,64,46>)
    n301 = Select(t=fxp<+,1,1> 0.0, s=w542, f=fxp<+,1,1> 1.0) -> (s? t:f=w539:fxp<+,1,1>)
    n302 = Add(x=w544, y=w537) -> (x+y=w543:fxp<+/-,32,16>)
    n303 = Multiply(x=w543, y=w539) -> (x*y=w538:fxp<+/-,32,16>)
    "Dy_i" <- w538
    n304 = call "Wait4"("Count(uSec)"=u32 1000) -> ()  [unwired: 1 out]
  }
  n305 = while "Encoder_y" {
    shift-right: [w577] -> _
    shift-left: _ -> [w575]
    shift-right: [w578] -> _
    shift-left: _ -> [w576]
    shift-right: [w581] -> _
    shift-left: _ -> [w580]
    stop <- FALSE stop-if-true
    n306 = xnode "FPGA I/O Node"() -> ("Mod4/DI0"=w582:bool, "Mod4/DI1"=w583:bool)  [unwired: 2 in, 2 out]
    n307 = call "encoder_sub.vi"("A_pre"=w575, "B_pre"=w576, "Encoder Position_pre"=w580, "A input"=w582, "Encoder Position Reset"="Encoder Reset_y", "B input"=w583) -> ("A"=w577:bool, "B"=w578:bool, "Encoder Position (Counts)"=w581:i32)  [unwired: 19 in]
    "Encoder Position_y" <- w581
    n308 = To Fixed-Point(number=w581) -> (fixed-point=w572:fxp<+/-,32,32>)  [unwired: 1 in]
    n309 = xnode "High Throughput Multiply"("x"=w572, "y"=fxp<+/-,24,0> 0.002499997615814209) -> ("x*y"=→"Dy (mm)":fxp<+/-,56,32>)
    n310 = xnode "High Throughput Multiply"("x"=w572, "y"=fxp<+/-,16,1> 0.125) -> ("x*y"=→"rad_y(NrTheta)":fxp<+/-,48,33>)
  }
  n311 = while "Command_y" {
    stop <- _ stop-if-true
    n312 = case shown="0, Default" "Command type_y" {
      tunnel: "Direction_y" -> [w588 _ _]
      tunnel: [w587 _ _] -> w584
      frame 0, Default {
        n313 = Select(s=w588) -> (s? t:f=w587:dbl)  [unwired: 2 in]
      }
      frame 1 {
      }
      frame 2 {
      }
    }
    "Dyr" <- w584
  }
